vi "_Insert Bundle Unbundle.vi"(7 "Block Diagram":refnum<vi>, 8 "error in (no error)":errorcluster, 11 "wires":refnum<vi>[](array[refnum])) -> (0 "error out":errorcluster, 3 "changes made?":bool)   [LabVIEW 2017]
doc: "把选中的多条 wire 按自上而下的位置顺序 Bundle 成一个 cluster，再 Unbundle 后接回原来的源端子与下游端子，数据流保持不变。\n\n限制：每根选中的 wire 只能有一个下游端子（无分叉）；有分叉时报错并放弃，不改动框图。\n\n输入：\nQD Launch VI Ref - QuickDrop 启动所在的 VI，取其 Block Diagram 的 Selection List[]（正常使用方式）。\nDiagnostic VI Path - 非空时改为打开该路径的 VI 并对该框图内所有 wire 操作，结束时保存该 VI（测试/批处理用）。\n\n输出：\nerror out - 选中对象不全是 wire、少于 2 根、或存在分叉时返回错误。\nchanges made? - 是否实际改动了框图。\n\nUndo 事务由调用方（QuickDrop 插件模板）管理。"
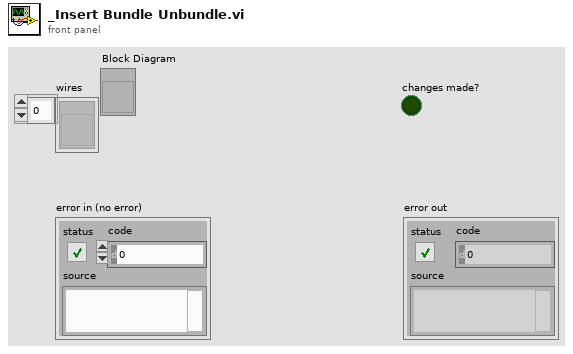
[diagram p1: front panel]
types:
  T1 = typedef "LVRectTypeDef.ctl" = cluster{"Left":i16, "Top":i16, "Right":i16, "Bottom":i16}
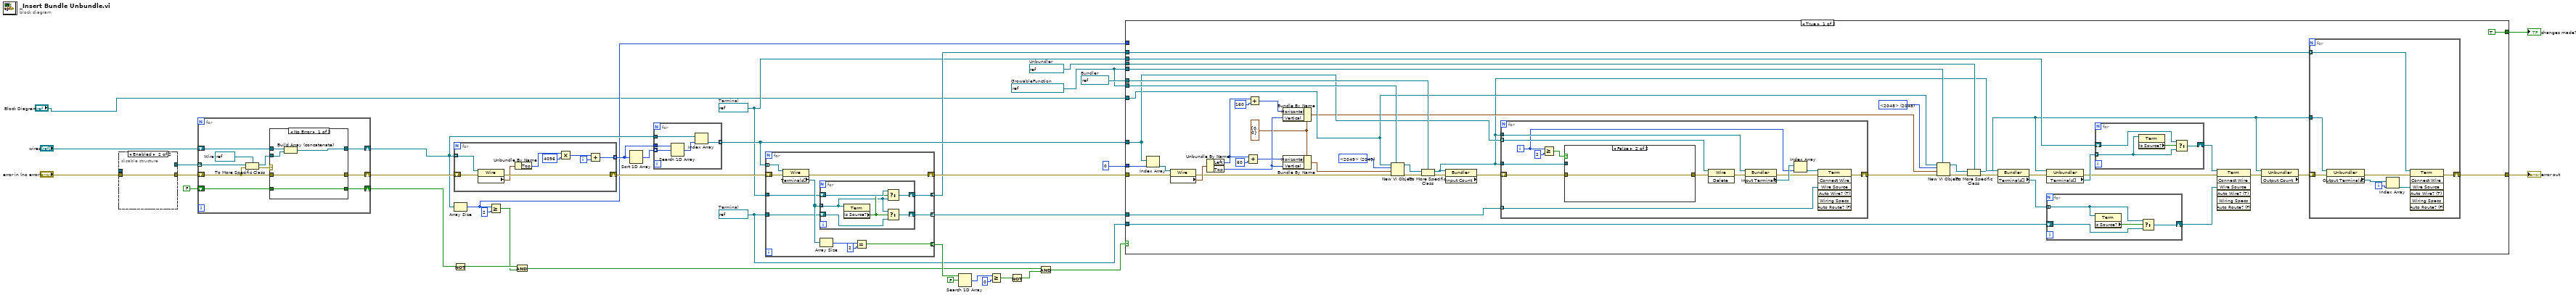
[diagram p0: block diagram]
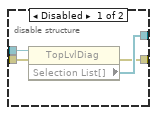
[diagram p2: hidden frame]
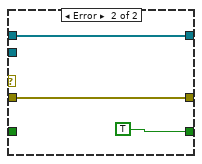
[diagram p3: hidden frame]
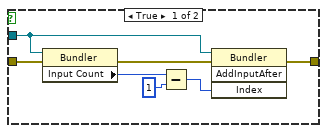
[diagram p4: hidden frame]
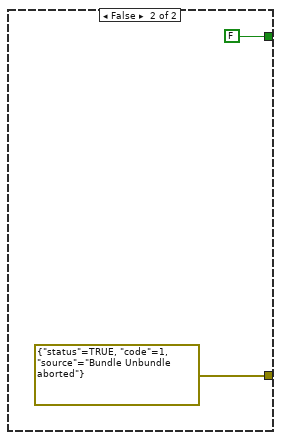
[diagram p5: hidden frame]
diagram:
  w7 = refnum<vi> refnum  # Terminal
  w8 = refnum<vi> refnum  # Terminal
  w10 = refnum<vi> refnum  # GrowableFunction
  w9 = refnum<vi> refnum  # Unbundler
  w11 = refnum<vi> refnum  # Bundler
  n1 = disable-structure shown="Enabled" {
    disable-tunnel: _ -> [w40 _]
    disable-tunnel: "error in (no error)" -> [w39 w41]
    disable-tunnel: [w38 _] -> w3
    disable-tunnel: [w37 w41] -> w2
    frame Disabled {
      n2 = property class="TopLvlDiag"(reference=w40, error in=w39) -> (error out=w37:errorcluster, "Selection List[]"=w38:refnum<vi>[])  [unwired: 1 out]
    }
    frame Enabled {
    }
  }
  n3 = for {
    tunnel: w3 -> [w51] mode=indexing
    shift-right: [w45] -> w24
    shift-left: "wires" -> [w48]
    shift-right: [w43] -> w33
    shift-left: w2 -> [w49]
    shift-right: [w44] -> w22
    shift-left: FALSE -> [w47]
    w50 = refnum<vi> refnum  # Wire
    n4 = To More Specific Class(target class=w50, reference=w51, error in=w49) -> (specific class reference=w46:refnum<vi>, error out=w42:errorcluster)
    n5 = case shown="No Error" w42 {
      tunnel: w49 -> [w55 w58]
      tunnel: w48 -> [w54 w59]
      tunnel: w47 -> [w56 _]
      tunnel: [w52 w59] -> w45
      tunnel: [w56 TRUE] -> w44
      tunnel: [w55 w58] -> w43
      tunnel: w46 -> [w53 _]
      frame No Error {
        n6 = Build Array (concatenate)(w54, w53) -> (w52:refnum<vi>[])
      }
      frame Error {
      }
    }
  }
  n7 = Not(x=w22) -> (.not. x?=w21:bool)
  n8 = for {
    tunnel: w24 -> [w68] mode=indexing
    tunnel: [w61] -> w31 mode=indexing
    shift-right: [w66] -> w30
    shift-left: w33 -> [w67]
    i -> [w60]
    n9 = property class="Wire"(reference=w68, error in=w67) -> (error out=w66:errorcluster, "Master Bounds Rect"=w65:T1)  [unwired: 1 out]
    n10 = Unbundle By Name(w65) -> ("Top"=w64:i16)
    n11 = Multiply(x=w64, y=4096) -> (x*y=w62:i32)
    n12 = Add(x=w62, y=w60) -> (x+y=w61:i32)
  }
  n13 = Array Size(array=w24) -> (size(s)=w15:i32)
  n14 = Greater Or Equal?(x=w15, y=2) -> (x >= y?=w20:bool)
  n15 = And(x=w21, y=w20) -> (x .and. y?=w19:bool)
  n16 = Sort 1D Array(array=w31) -> (sorted array=w32:i32[])
  n17 = for {
    tunnel: w32 -> [w72] mode=indexing
    tunnel: w31 -> [w73]
    tunnel: w24 -> [w71]
    tunnel: [w69] -> w16 mode=indexing
    n18 = Search 1D Array(1D array=w73, element=w72) -> (index of element=w70:i32)  [unwired: 1 in]
    n19 = Index Array(array=w71, index=w70) -> (element=w69:refnum<vi>)
  }
  n20 = for {
    tunnel: w16 -> [w84] mode=indexing
    shift-right: [w82] -> w17
    shift-left: w30 -> [w83]
    tunnel: [w79] -> w29 mode=indexing
    tunnel: [w77] -> w14 mode=indexing
    tunnel: [w75] -> w13 mode=indexing
    tunnel: w8 -> [w76]
    tunnel: w7 -> [w74]
    n21 = property class="Wire"(reference=w84, error in=w83) -> (error out=w82:errorcluster, "Terminals[]"=w78:refnum<vi>[])  [unwired: 1 out]
    n22 = for {
      tunnel: w78 -> [w86] mode=indexing
      shift-right: [w89] -> w77
      shift-left: w76 -> [w90]
      shift-right: [w85] -> w75
      shift-left: w74 -> [w88]
      n23 = property class="Term"(reference=w86) -> ("Is Source?"=w87:bool)  [unwired: 1 in, 2 out]
      n24 = Select(t=w88, s=w87, f=w86) -> (s? t:f=w85:refnum<vi>)
      n25 = Select(t=w86, s=w87, f=w90) -> (s? t:f=w89:refnum<vi>)
    }
    n26 = Array Size(array=w78) -> (size(s)=w81:i32)
    n27 = Equal?(x=w81, y=2) -> (x = y?=w79:bool)
  }
  n28 = Search 1D Array(1D array=w29, element=FALSE) -> (index of element=w27:i32)  [unwired: 1 in]
  n29 = Greater Or Equal?(x=w27, y=0) -> (x >= y?=w25:bool)
  n30 = Not(x=w25) -> (.not. x?=w18:bool)
  n31 = And(x=w19, y=w18) -> (x .and. y?=w5:bool)
  n32 = case shown="True" w5 {
    tunnel: w17 -> [w133 _]
    tunnel: w16 -> [w116 _]
    tunnel: w15 -> [_ _]
    tunnel: "Block Diagram" -> [w113 _]
    tunnel: w14 -> [w115 _]
    tunnel: w13 -> [w94 _]
    tunnel: [w93 errorcluster {"status"=TRUE, "code"=1, "source"="Bundle Unbundle aborted"}] -> w4
    tunnel: [TRUE FALSE] -> w6
    tunnel: 0 -> [w135 _]
    tunnel: w10 -> [w121 _]
    tunnel: w11 -> [w118 _]
    tunnel: w10 -> [w109 _]
    tunnel: w9 -> [w106 _]
    tunnel: w8 -> [w102 _]
    tunnel: w7 -> [w99 _]
    frame True {
      w112 = 2048 items=[""=2041, "<2048>"=2048, "<2049>"=2049]
      w124 = 2049 items=[""=2041, "<2048>"=2048, "<2049>"=2049]
      w125 = cluster{"Horizontal":i16, "Vertical":i16} {"Horizontal"=0, "Vertical"=0}
      n33 = Index Array(array=w116, index=w135) -> (element=w134:refnum<vi>)
      n34 = property class="Wire"(reference=w134, error in=w133) -> (error out=w122:errorcluster, "Master Bounds Rect"=w132:T1)  [unwired: 1 out]
      n35 = Unbundle By Name(w132) -> ("Left"=w130:i16, "Top"=w126:i16)
      n36 = Add(x=w130, y=60) -> (x+y=w128:i32)
      n37 = Add(x=w130, y=160) -> (x+y=w127:i32)
      n38 = Bundle By Name(cluster=w125, "Horizontal"=w127, "Vertical"=w126) -> (w111:cluster{"Horizontal":i16, "Vertical":i16})
      n39 = Bundle By Name(cluster=w125, "Horizontal"=w128, "Vertical"=w126) -> (w123:cluster{"Horizontal":i16, "Vertical":i16})
      n40 = New VI Object(vi object class=w121, owner refnum=w113, style=w124, position/next to=w123, 8:w122) -> (object refnum=w120:refnum<vi>, 0:w119:errorcluster)  [unwired: 3 in]
      n41 = To More Specific Class(target class=w118, reference=w120, error in=w119) -> (specific class reference=w105:refnum<vi>, error out=w117:errorcluster)
      n42 = property class="Bundler" props=["Input Count"](reference=w105, error in=w117) -> (error out=w114:errorcluster)  [unwired: 2 out]
      n43 = for {
        tunnel: w116 -> [w162] mode=indexing
        tunnel: w115 -> [w155] mode=indexing
        shift-right: [w154] -> w110
        shift-left: w114 -> [w165]
        tunnel: w105 -> [w164]
        tunnel: w105 -> [w160]
        i -> [w153]
        n44 = Greater Or Equal?(x=w153, y=2) -> (x >= y?=w163:bool)
        n45 = case shown="False" w163 {
          tunnel: w165 -> [w173 w174]
          tunnel: w164 -> [w170 _]
          tunnel: [w167 w174] -> w161
          frame True {
            n46 = property class="Bundler"(reference=w170, error in=w173) -> (error out=w169:errorcluster, "Input Count"=w172:i32)  [unwired: 1 out]
            n47 = Subtract(x=w172, y=1) -> (x-y=w168:i32)
            n48 = invoke class="Bundler" method="AddInputAfter"(reference=w170, error in=w169, "Index"=w168) -> (error out=w167:errorcluster)  [unwired: 1 in, 3 out]
          }
          frame False {
          }
        }
        n49 = invoke class="Wire" method="Delete"(reference=w162, error in=w161) -> (error out=w159:errorcluster)  [unwired: 1 in, 2 out]
        n50 = property class="Bundler"(reference=w160, error in=w159) -> (error out=w156:errorcluster, "Input Terminals"=w158:refnum<vi>[])  [unwired: 1 out]
        n51 = Index Array(array=w158, index=w153) -> (element=w157:refnum<vi>)
        n52 = invoke class="Term" method="Connect Wire"(reference=w157, error in=w156, "Wire Source"=w155) -> (error out=w154:errorcluster)  [unwired: 4 in, 6 out]
      }
      n53 = New VI Object(vi object class=w109, owner refnum=w113, style=w112, position/next to=w111, 8:w110) -> (object refnum=w108:refnum<vi>, 0:w107:errorcluster)  [unwired: 3 in]
      n54 = To More Specific Class(target class=w106, reference=w108, error in=w107) -> (specific class reference=w91:refnum<vi>, error out=w104:errorcluster)
      n55 = property class="Bundler"(reference=w105, error in=w104) -> (error out=w101:errorcluster, "Terminals[]"=w103:refnum<vi>[])  [unwired: 1 out]
      n56 = property class="Unbundler"(reference=w91, error in=w101) -> (error out=w97:errorcluster, "Terminals[]"=w100:refnum<vi>[])  [unwired: 1 out]
      n57 = for {
        tunnel: w103 -> [w152] mode=indexing
        shift-right: [w149] -> w96
        shift-left: w102 -> [w150]
        n58 = property class="Term"(reference=w152) -> ("Is Source?"=w151:bool)  [unwired: 1 in, 2 out]
        n59 = Select(t=w152, s=w151, f=w150) -> (s? t:f=w149:refnum<vi>)
      }
      n60 = for {
        tunnel: w100 -> [w146] mode=indexing
        shift-right: [w145] -> w98
        shift-left: w99 -> [w148]
        n61 = property class="Term"(reference=w146) -> ("Is Source?"=w147:bool)  [unwired: 1 in, 2 out]
        n62 = Select(t=w148, s=w147, f=w146) -> (s? t:f=w145:refnum<vi>)
      }
      n63 = invoke class="Term" method="Connect Wire"(reference=w98, error in=w97, "Wire Source"=w96) -> (error out=w95:errorcluster)  [unwired: 4 in, 6 out]
      n64 = property class="Unbundler" props=["Output Count"](reference=w91, error in=w95) -> (error out=w92:errorcluster)  [unwired: 2 out]
      n65 = for {
        tunnel: w94 -> [w141] mode=indexing
        shift-right: [w138] -> w93
        shift-left: w92 -> [w143]
        tunnel: w91 -> [w144]
        i -> [w137]
        n66 = property class="Unbundler"(reference=w144, error in=w143) -> (error out=w140:errorcluster, "Output Terminals[]"=w142:refnum<vi>[])  [unwired: 1 out]
        n67 = Index Array(array=w142, index=w137) -> (element=w139:refnum<vi>)
        n68 = invoke class="Term" method="Connect Wire"(reference=w141, error in=w140, "Wire Source"=w139) -> (error out=w138:errorcluster)  [unwired: 4 in, 6 out]
      }
    }
    frame False {
    }
  }
  "changes made?" <- w6
  "error out" <- w4
